vi "Temperatur Anpassen.vi"(0 "Verbindungs-ID In":refnum<k16>, 5 "Soll-Temperatur":dbl, 7 "Ist-Temperatur":dbl, 9 "Thermostat in %":dbl, 11 "Fehler (Eingang)":errorcluster) -> (4 "Verbindungs-ID-Out":refnum<k16>, 10 "Neuer Thermostat-Wert in %":dbl, 15 "Fehler (Ausgang)":errorcluster)   [LabVIEW 2024]
doc: "Passt das Ventil des Thermostats an. Die Verbindungs-ID ist die UDP-Verbindung zum Thermostat. Soll- und Ist-Temperatur geben die gewünschte und die aktuelle Temperatur des Heizkörpers an."
uses:
  <vilib>/addons/control/pid/NI_PID_pid.lvlib
  Treiber Heizung/Thermostat Treiber.lvlib
  <vilib>/addons/control/pid/pid.llb/PID (DBL).vi
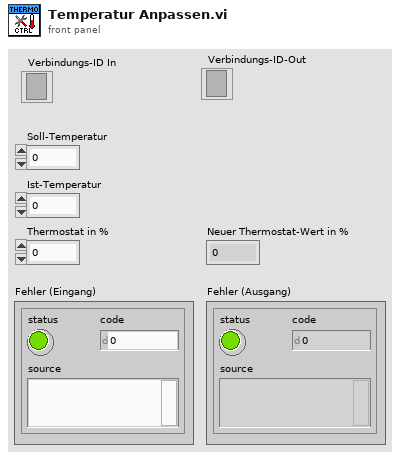
[diagram p1: front panel]
types:
  T1 = cluster{"proportional gain (Kc)":dbl, "integral time (Ti, min)":dbl, "derivative time (Td, min)":dbl}
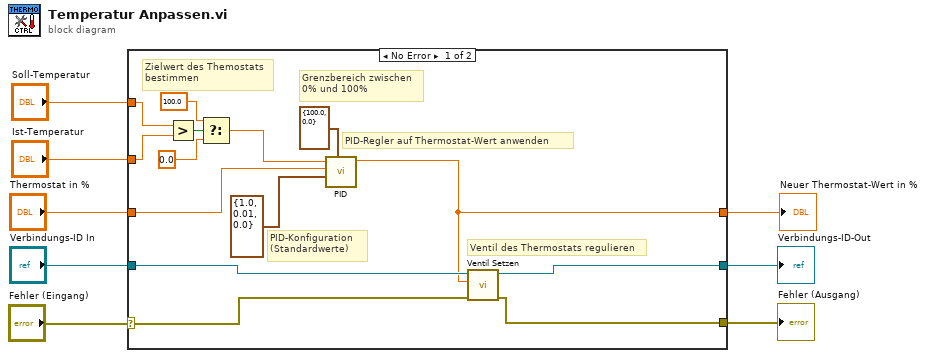
[diagram p0: block diagram]
diagram:
  n1 = case shown="No Error" "Fehler (Eingang)" {
    selector: "Fehler (Eingang)" -> [w19 w25]
    tunnel: [w18 w25] -> w7
    tunnel: "Verbindungs-ID In" -> [w20 w24]
    tunnel: [w17 w24] -> w5
    tunnel: "Ist-Temperatur" -> [w12 _]
    tunnel: "Soll-Temperatur" -> [w13 _]
    tunnel: "Thermostat in %" -> [w16 w23]
    tunnel: [w15 w23] -> w1
    frame No Error {
      # "Zielwert des Themostats\nbestimmen"
      # "Ventil des Thermostats regulieren"
      # "PID-Konfiguration\n(Standardwerte)"
      # "PID-Regler auf Thermostat-Wert anwenden"
      # "Grenzbereich zwischen\n0% und 100%"
      n2 = Greater?(x=w13, y=w12) -> (0:w14:bool)
      n3 = Select(t=100.0, s=w14, f=0.0) -> (s? t:f=w11:dbl)
      n4 = call-poly <vilib>:"PID.vi"("output range"=cluster{"output high":dbl, "output low":dbl} {"output high"=100.0, "output low"=0.0}, "PID gains"=T1 {"proportional gain (Kc)"=1.0, "integral time (Ti, min)"=0.01, "derivative time (Td, min)"=0.0}, "process variable"=w16, "setpoint"=w11) -> ("output"=w15:dbl)  [unwired: 6 in, 1 out]
      n5 = call "Ventil Setzen.vi"("Error In"=w19, "Thermostat in %"=w15, "Verbindungs-ID in"=w20) -> ("Error Out"=w18:errorcluster, "Verbindungs-ID out"=w17:refnum<k16>)  [unwired: 7 in]
    }
    frame Error {
    }
  }
  "Fehler (Ausgang)" <- w7
  "Verbindungs-ID-Out" <- w5
  "Neuer Thermostat-Wert in %" <- w1
